vi "myRIO_BRig_RT__Case_Exp_State_initTrial_LC_Sel__v2.vi"(6 "input_dataTrial":u16[][](array[numeric]), 7 "input_spout":enum16{"Left", "Right"}(ring), 9 "input_dataBlock":u16[][](array[numeric]), 10 "input_dataLC":u16[](array[numeric]), 11 "input_dataCurrent":u16[](array[numeric])) -> (2 "output_LC__Sel":bool, 3 "output_LC_led__Sel":bool, 4 "output_dataTrial":u16[][](array[numeric]), 5 "output_dataCurrent":u16[](array[numeric]))   [LabVIEW 2014]
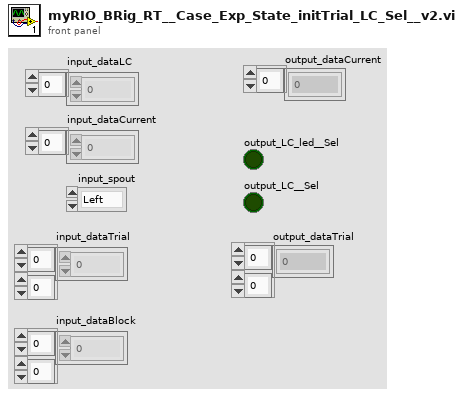
[diagram p1: front panel]
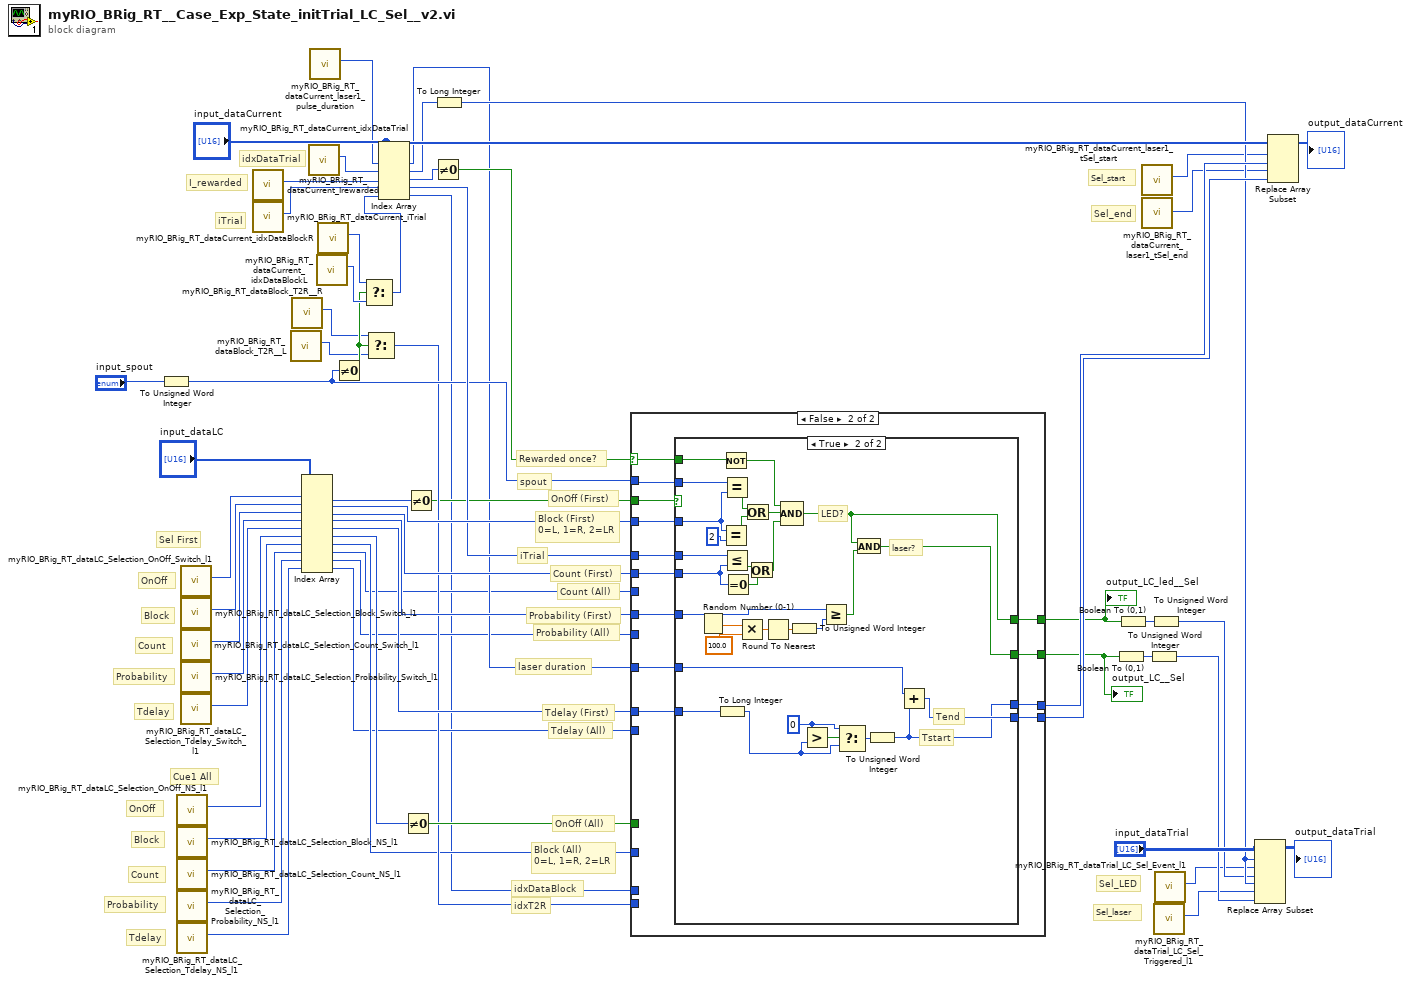
[diagram p0: block diagram]
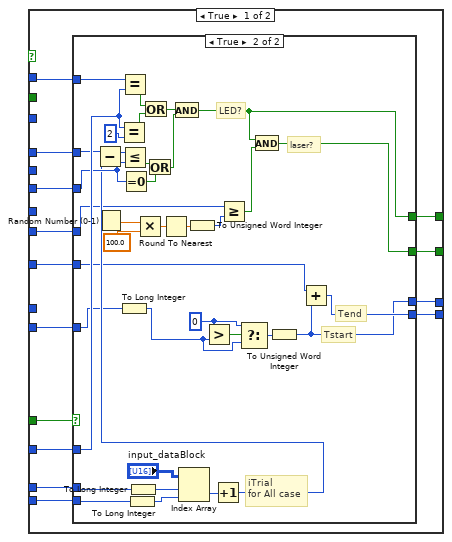
[diagram p2: hidden frame]
diagram:
  # "Tdelay (All)"
  # "Probability (All)"
  # "Count (All)"
  # "Block (All)\n0=L, 1=R, 2=LR"
  # "idxT2R"
  # "idxDataBlock"
  # "OnOff (All)"
  # "Count"
  # "Tdelay"
  # "Probability"
  # "OnOff"
  # "Block"
  # "Cue1 All"
  # "Tdelay (First)"
  # "laser duration"
  # "Probability (First)"
  # "Count (First)"
  # "iTrial"
  # "Block (First)\n0=L, 1=R, 2=LR"
  # "spout"
  # "Rewarded once?"
  # "OnOff (First)"
  # "iTrial"
  # "Sel_LED"
  # "Sel_laser"
  # "idxDataTrial"
  # "Sel_end"
  # "Sel_start"
  # "Tdelay"
  # "I_rewarded"
  # "Sel First"
  # "Probability"
  # "Count"
  # "Block"
  # "OnOff"
  n1 = To Unsigned Word Integer(number="input_spout") -> (unsigned 16bit integer=w32:u16)
  n2 = call "myRIO_BRig_RT_dataLC_Selection_OnOff_NS_l1.vi"() -> ("output_Selection_OnOff_NS_l1"=w11:i32)  [unwired: 11 in]
  n3 = call "myRIO_BRig_RT_dataLC_Selection_Block_NS_l1.vi"() -> ("output_Selection_Block_NS_l1"=w10:i32)  [unwired: 11 in]
  n4 = call "myRIO_BRig_RT_dataLC_Selection_Count_NS_l1.vi"() -> ("output_Selection_Count_NS_l1"=w9:i32)  [unwired: 11 in]
  n5 = call "myRIO_BRig_RT_dataLC_Selection_Probability_NS_l1.vi"() -> ("output_Selection_Probability_NS_l1"=w8:i32)  [unwired: 11 in]
  n6 = call "myRIO_BRig_RT_dataLC_Selection_Tdelay_NS_l1.vi"() -> ("output_Selection_Tdelay_NS_l1"=w7:i32)  [unwired: 11 in]
  n7 = call "myRIO_BRig_RT_dataLC_Selection_OnOff_Switch_l1.vi"() -> ("output_Selection_OnOff_Switch_l1"=w21:i32)  [unwired: 11 in]
  n8 = call "myRIO_BRig_RT_dataLC_Selection_Block_Switch_l1.vi"() -> ("output_Selection_Block_Switch_l1"=w20:i32)  [unwired: 11 in]
  n9 = call "myRIO_BRig_RT_dataLC_Selection_Count_Switch_l1.vi"() -> ("output_Selection_Count_Switch_l1"=w19:i32)  [unwired: 11 in]
  n10 = call "myRIO_BRig_RT_dataLC_Selection_Probability_Switch_l1.vi"() -> ("output_Selection_Probability_Switch_l1"=w18:i32)  [unwired: 11 in]
  n11 = call "myRIO_BRig_RT_dataLC_Selection_Tdelay_Switch_l1.vi"() -> ("output_Selection_Tdelay_Switch_l1"=w17:i32)  [unwired: 11 in]
  n12 = call "myRIO_BRig_RT_dataCurrent_Irewarded.vi"() -> ("output_I_rewarded"=w52:i32)  [unwired: 11 in]
  n13 = call "myRIO_BRig_RT_dataCurrent_iTrial.vi"() -> ("output_iTrial"=w35:i32)  [unwired: 11 in]
  n14 = call "myRIO_BRig_RT_dataBlock_T2R__L.vi"() -> ("output_T2R__L"=w27:i32)  [unwired: 11 in]
  n15 = call "myRIO_BRig_RT_dataBlock_T2R__R.vi"() -> ("output_T2R__R"=w28:i32)  [unwired: 11 in]
  n16 = Index Array(array="input_dataLC", index #1=w21, index #2=w20, index #3=w19, index #4=w18, index #5=w17, index #6=w11, index #7=w10, index #8=w9, index #9=w8, index #10=w7) -> (element #1=w58:u16, element #2=w55:u16, element #3=w56:u16, element #4=w57:u16, element #5=w51:u16, element #6=w16:u16, element #7=w15:u16, element #8=w14:u16, element #9=w13:u16, element #10=w12:u16)
  n17 = call "myRIO_BRig_RT_dataCurrent_idxDataTrial.vi"() -> ("output_idxDataTrial"=w40:i32)  [unwired: 11 in]
  n18 = call "myRIO_BRig_RT_dataCurrent_laser1_pulse_duration.vi"() -> ("output_laser1_pulse_duration"=w23:i32)  [unwired: 11 in]
  n19 = call "myRIO_BRig_RT_dataCurrent_idxDataBlockL.vi"() -> ("output_idxDataBlock__L"=w31:i32)  [unwired: 11 in]
  n20 = call "myRIO_BRig_RT_dataCurrent_idxDataBlockR.vi"() -> ("output_idxDataBlock__R"=w30:i32)  [unwired: 11 in]
  n21 = Not Equal To 0?(x=w32) -> (x != 0?=w29:bool)
  n22 = Select(t=w30, s=w29, f=w31) -> (s? t:f=w6:i32)
  n23 = Select(t=w28, s=w29, f=w27) -> (s? t:f=w26:i32)
  n24 = Index Array(array="input_dataCurrent", index #1=w23, index #2=w40, index #3=w52, index #4=w35, index #5=w6) -> (element #1=w22:u16, element #2=w39:u16, element #3=w53:u16, element #4=w34:u16, element #5=w5:u16)
  n25 = Not Equal To 0?(x=w16) -> (x != 0?=w33:bool)
  n26 = Not Equal To 0?(x=w58) -> (x != 0?=w24:bool)
  n27 = Not Equal To 0?(x=w53) -> (x != 0?=w25:bool)
  n28 = To Long Integer(number=w39) -> (32bit integer=w38:i32)
  n29 = case shown="False" w25 {
    selector: w25 -> [_ w111]
    tunnel: w55 -> [_ w121]
    tunnel: w56 -> [_ w113]
    tunnel: w57 -> [_ w119]
    tunnel: [w70 w117] -> w43
    tunnel: [w71 w118] -> w45
    tunnel: w32 -> [w73 w122]
    tunnel: w51 -> [_ w115]
    tunnel: w22 -> [w67 w112]
    tunnel: [w68 w114] -> w48
    tunnel: [w69 w116] -> w47
    tunnel: w34 -> [w72 w120]
    tunnel: w33 -> [w60 _]
    tunnel: w26 -> [w66 _]
    tunnel: w5 -> [w65 _]
    tunnel: w15 -> [w64 _]
    tunnel: w14 -> [w63 _]
    tunnel: w13 -> [w62 _]
    tunnel: w12 -> [w61 _]
    tunnel: w24 -> [_ w110]
    frame True {
      n30 = case shown="True" w60 {
        tunnel: w73 -> [_ w108]
        tunnel: w72 -> [_ w87]
        tunnel: [_ w82] -> w71
        tunnel: [_ w99] -> w70
        tunnel: [_ w78] -> w69
        tunnel: [_ w77] -> w68
        tunnel: w67 -> [_ w76]
        tunnel: w66 -> [_ w93]
        tunnel: w65 -> [_ w95]
        tunnel: w64 -> [_ w90]
        tunnel: w63 -> [_ w89]
        tunnel: w62 -> [_ w85]
        tunnel: w61 -> [_ w75]
        frame False {
        }
        frame True {
          w80 = 0 ("x")
          # "Tstart"
          # "Tend"
          # "iTrial\nfor All case"
          # "laser?"
          # "LED?"
          n31 = Random Number (0-1)() -> (number: 0 to 1=w105:dbl)
          n32 = Equal?(x=w90, y=u16 2) -> (x = y?=w106:bool)
          n33 = To Long Integer(number=w75) -> (32bit integer=w74:i32)
          n34 = Equal?(x=w108, y=w90) -> (x = y?=w107:bool)
          n35 = Equal To 0?(x=w89) -> (x = 0?=w97:bool)
          n36 = To Long Integer(number=w93) -> (32bit integer=w92:i32)
          n37 = To Long Integer(number=w95) -> (32bit integer=w94:i32)
          n38 = Multiply(x=w105, y=100.0) -> (x*y=w104:dbl)
          n39 = Or(x=w107, y=w106) -> (x .or. y?=w84:bool)
          n40 = Round To Nearest(number=w104) -> (nearest integer value=w103:dbl)
          n41 = Index Array(array="input_dataBlock", index (row)=w94, index (col)=w92) -> (element=w91:u16)
          n42 = To Unsigned Word Integer(number=w103) -> (unsigned 16bit integer=w101:u16)
          n43 = Greater?(x=w80, y=w74) -> (0:w79:bool)
          n44 = Increment(x=w91) -> (x+1=w88:u16)
          n45 = Subtract(x=w87, y=w88) -> (x-y=w86:u16)
          n46 = Less Or Equal?(x=w86, y=w89) -> (x <= y?=w98:bool)
          n47 = Or(x=w98, y=w97) -> (x .or. y?=w83:bool)
          n48 = And(x=w84, y=w83) -> (x .and. y?=w82:bool)
          n49 = Greater Or Equal?(x=w85, y=w101) -> (x >= y?=w100:bool)
          n50 = Select(t=w80, s=w79, f=w74) -> (s? t:f=w81:i32)
          n51 = And(x=w82, y=w100) -> (x .and. y?=w99:bool)
          n52 = To Unsigned Word Integer(number=w81) -> (unsigned 16bit integer=w77:u16)
          n53 = Add(x=w76, y=w77) -> (x+y=w78:u16)
        }
      }
    }
    frame False {
      n54 = case shown="True" w110 {
        tunnel: w122 -> [_ w151]
        tunnel: w121 -> [_ w150]
        tunnel: w120 -> [_ w149]
        tunnel: w119 -> [_ w142]
        tunnel: [_ w137] -> w118
        tunnel: [_ w136] -> w117
        tunnel: [_ w125] -> w116
        tunnel: w115 -> [_ w127]
        tunnel: [_ w124] -> w114
        tunnel: w113 -> [_ w135]
        tunnel: w112 -> [_ w126]
        tunnel: w111 -> [_ w131]
        frame False {
        }
        frame True {
          w129 = 0 ("x")
          # "Tstart"
          # "Tend"
          # "laser?"
          # "LED?"
          n55 = Random Number (0-1)() -> (number: 0 to 1=w146:dbl)
          n56 = To Long Integer(number=w127) -> (32bit integer=w123:i32)
          n57 = Not(x=w131) -> (.not. x?=w140:bool)
          n58 = Equal?(x=w150, y=u16 2) -> (x = y?=w147:bool)
          n59 = Equal?(x=w151, y=w150) -> (x = y?=w148:bool)
          n60 = Less Or Equal?(x=w149, y=w135) -> (x <= y?=w134:bool)
          n61 = Equal To 0?(x=w135) -> (x = 0?=w133:bool)
          n62 = Multiply(x=w146, y=100.0) -> (x*y=w145:dbl)
          n63 = Or(x=w148, y=w147) -> (x .or. y?=w139:bool)
          n64 = Or(x=w134, y=w133) -> (x .or. y?=w132:bool)
          n65 = Round To Nearest(number=w145) -> (nearest integer value=w144:dbl)
          n66 = Compound Arithmetic op=AND(w140, w139, w132) -> (w137:bool)
          n67 = To Unsigned Word Integer(number=w144) -> (unsigned 16bit integer=w141:u16)
          n68 = Greater?(x=w129, y=w123) -> (0:w128:bool)
          n69 = Greater Or Equal?(x=w142, y=w141) -> (x >= y?=w138:bool)
          n70 = Select(t=w129, s=w128, f=w123) -> (s? t:f=w130:i32)
          n71 = And(x=w137, y=w138) -> (x .and. y?=w136:bool)
          n72 = To Unsigned Word Integer(number=w130) -> (unsigned 16bit integer=w124:u16)
          n73 = Add(x=w126, y=w124) -> (x+y=w125:u16)
        }
      }
    }
  }
  "output_LC__Sel" <- w43
  "output_LC_led__Sel" <- w45
  n74 = Boolean To (0,1)(Boolean=w43) -> (0, 1=w44:i16)
  n75 = Boolean To (0,1)(Boolean=w45) -> (0, 1=w46:i16)
  n76 = call "myRIO_BRig_RT_dataCurrent_laser1_tSel_start.vi"() -> ("output_laser1_tSel_start"=w4:i32)  [unwired: 11 in]
  n77 = call "myRIO_BRig_RT_dataCurrent_laser1_tSel_end.vi"() -> ("output_laser1_tSel_end"=w3:i32)  [unwired: 11 in]
  n78 = To Unsigned Word Integer(number=w44) -> (unsigned 16bit integer=w36:u16)
  n79 = To Unsigned Word Integer(number=w46) -> (unsigned 16bit integer=w37:u16)
  n80 = call "myRIO_BRig_RT_dataTrial_LC_Sel_Triggered_l1.vi"() -> ("output_LC_Sel_Triggered_l1"=w1:i32)  [unwired: 11 in]
  n81 = call "myRIO_BRig_RT_dataTrial_LC_Sel_Event_l1.vi"() -> ("output_LC_Sel_Event_l1"=w2:i32)  [unwired: 11 in]
  n82 = Replace Array Subset(array="input_dataTrial", new element #1=w37, index (row) #1=w38, index (col) #1=w2, new element #2=w36, index (row) #2=w38, index (col) #2=w1) -> (→"output_dataTrial":u16[][])
  n83 = Replace Array Subset(array="input_dataCurrent", new element #1=w48, index #1=w4, new element #2=w47, index #2=w3) -> (→"output_dataCurrent":u16[])
